vi "力特性判定.vi"(0 "曲线引用":refnum<vi>, 1 "力特性":T1, 3 "错误输入":errorcluster) -> (7 "曲线引用输出":refnum<vi>, 8 "OK？":bool, 10 "错误输出":errorcluster)   [LabVIEW 2018]
uses:
  Global_Variable/Global.vi
  Global_Variable/A180648.vi
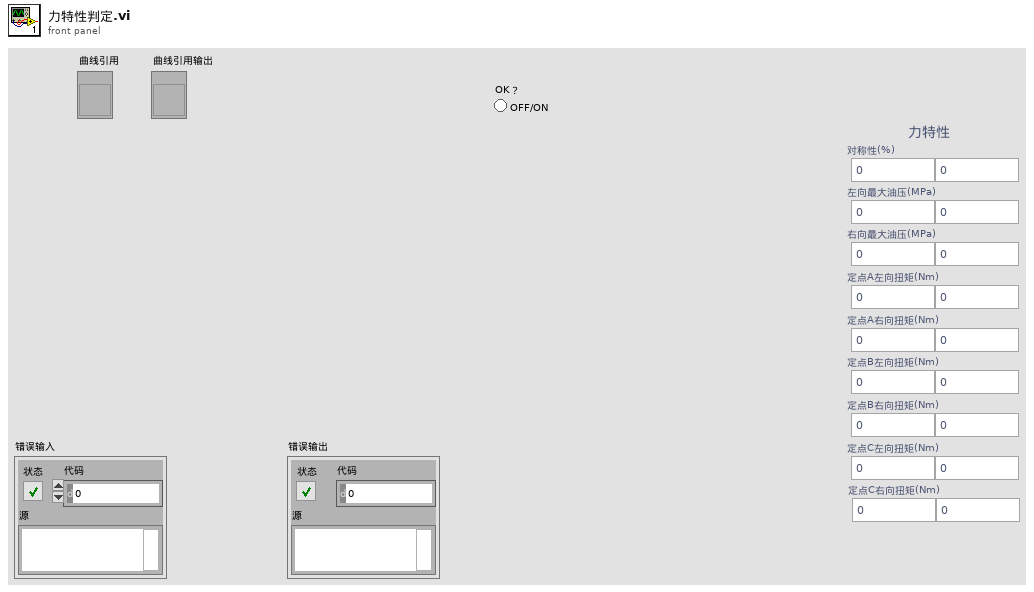
[diagram p1: front panel]
types:
  T1 = cluster{"对称性(%)":cluster{"下限":dbl, "上限":dbl}, "左向最大油压(MPa)":cluster{"下限":dbl, "上限":dbl}, "右向最大油压(MPa)":cluster{"下限":dbl, "上限":dbl}, "定点A左向扭矩(Nm)":cluster{"下限":dbl, "上限":dbl}, "定点A右向扭矩(Nm)":cluster{"下限":dbl, "上限":dbl}, "定点B左向扭矩(Nm)":cluster{"下限":dbl, "上限":dbl}, "定点B右向扭矩(Nm)":cluster{"下限":dbl, "上限":dbl}, "定点C左向扭矩(Nm)":cluster{"下限":dbl, "上限":dbl}, "定点C右向扭矩(Nm)":cluster{"下限":dbl, "上限":dbl}}
  T2 = enum32{"空载", "功能", "力特性", "传感器特性", "电流特性", "振动NVH", "逆向空载", "完成"}
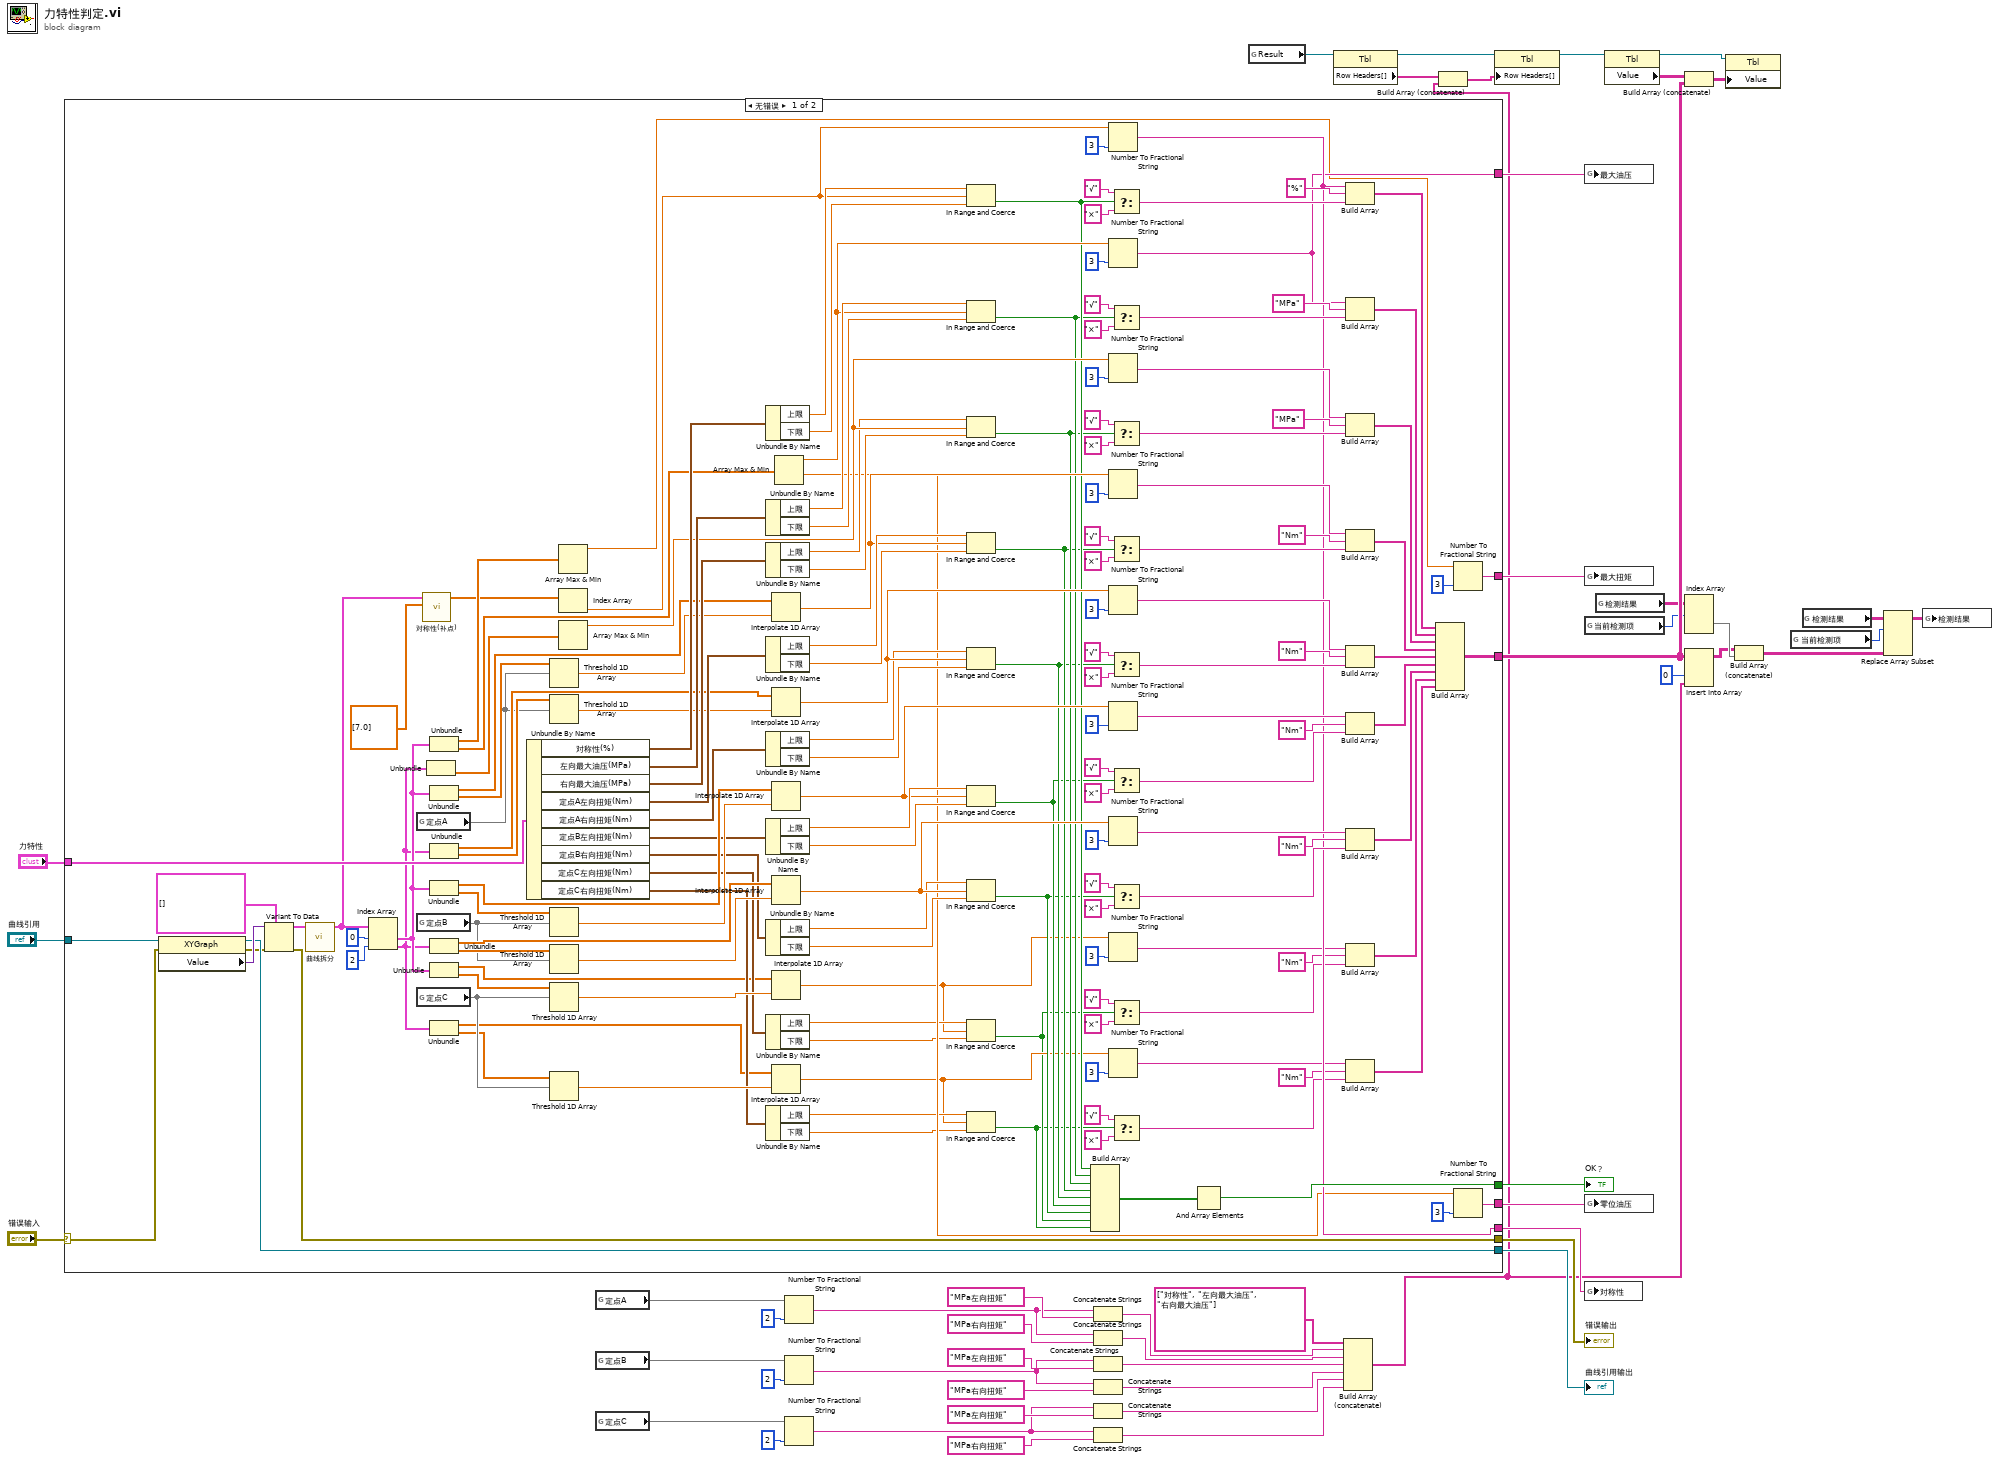
[diagram p0: block diagram]
diagram:
  n1 = case shown="无错误" "错误输入" {
    selector: "错误输入" -> [w206 w210]
    tunnel: [w203 w210] -> w50
    tunnel: "曲线引用" -> [w202 w209]
    tunnel: [w205 w209] -> w48
    tunnel: [w104 _] -> w47
    tunnel: "力特性" -> [w201 _]
    tunnel: [w103 _] -> w10
    tunnel: [w98 _] -> w25
    tunnel: [w97 _] -> w24
    tunnel: [w93 _] -> w23
    tunnel: [w90 _] -> w22
    frame No Error {
      n2 = property class="XYGraph"(reference=w202, error in=w206) -> (reference out=w205:refnum<vi>, error out=w204:errorcluster, "Value"=w208:variant)
      n3 = Variant To Data(error in=w204, type=cluster{dbl[], dbl[]}[] [], Variant=w208) -> (data=w56:cluster{dbl[], dbl[]}[], error out=w203:errorcluster)
      n4 = call "曲线拆分.vi"("原始曲线"=w56) -> ("拆分后曲线"=w55:cluster{dbl[], dbl[]}[])  [unwired: 10 in]
      n5 = Index Array(array=w55, index #1=0 ("索引"), index #2=2 ("索引")) -> (element #1=w70:cluster{dbl[], dbl[]}, element #2=w69:cluster{dbl[], dbl[]})
      n6 = global read "A180648.vi" "定点A"() -> (w100)
      n7 = global read "A180648.vi" "定点B"() -> (w99)
      n8 = global read "A180648.vi" "定点C"() -> (w65)
      n9 = call "对称性(补点).vi"("检测点"=dbl[] [7.0], "XY图"=w55) -> ("对称性"=w53:dbl[])  [unwired: 9 in]
      n10 = Unbundle(w69) -> (w101:dbl[])  [unwired: 1 out]
      n11 = Unbundle(w70) -> (w96:dbl[], w102:dbl[])
      n12 = Unbundle(w70) -> (w164:dbl[], w165:dbl[])
      n13 = Unbundle(w69) -> (w158:dbl[], w157:dbl[])
      n14 = Unbundle(w70) -> (w138:dbl[], w139:dbl[])
      n15 = Unbundle(w69) -> (w130:dbl[], w129:dbl[])
      n16 = Unbundle(w70) -> (w61:dbl[], w66:dbl[])
      n17 = Unbundle(w69) -> (w62:dbl[], w64:dbl[])
      n18 = Unbundle By Name(w201) -> ("对称性(%)"=w200:cluster{"下限":dbl, "上限":dbl}, "左向最大油压(MPa)"=w185:cluster{"下限":dbl, "上限":dbl}, "右向最大油压(MPa)"=w174:cluster{"下限":dbl, "上限":dbl}, "定点A左向扭矩(Nm)"=w161:cluster{"下限":dbl, "上限":dbl}, "定点A右向扭矩(Nm)"=w148:cluster{"下限":dbl, "上限":dbl}, "定点B左向扭矩(Nm)"=w133:cluster{"下限":dbl, "上限":dbl}, "定点B右向扭矩(Nm)"=w120:cluster{"下限":dbl, "上限":dbl}, "定点C左向扭矩(Nm)"=w68:cluster{"下限":dbl, "上限":dbl}, "定点C右向扭矩(Nm)"=w67:cluster{"下限":dbl, "上限":dbl})
      n19 = Threshold 1D Array(2:w100, 3:w165) -> (0:w163:dbl)  [unwired: 1 in]
      n20 = Threshold 1D Array(2:w100, 3:w157) -> (0:w159:dbl)  [unwired: 1 in]
      n21 = Threshold 1D Array(2:w99, 3:w139) -> (0:w137:dbl)  [unwired: 1 in]
      n22 = Threshold 1D Array(2:w99, 3:w129) -> (0:w131:dbl)  [unwired: 1 in]
      n23 = Threshold 1D Array(2:w65, 3:w66) -> (0:w71:dbl)  [unwired: 1 in]
      n24 = Threshold 1D Array(2:w65, 3:w64) -> (0:w81:dbl)  [unwired: 1 in]
      n25 = Array Max & Min(array=w96) -> (max value=w94:dbl)  [unwired: 3 out]
      n26 = Index Array(array=w53) -> (element=w52:dbl)  [unwired: 1 in]
      n27 = Array Max & Min(array=w101) -> (max value=w183:dbl)  [unwired: 3 out]
      n28 = Unbundle By Name(w200) -> ("上限"=w199:dbl, "下限"=w198:dbl)
      n29 = Unbundle By Name(w185) -> ("上限"=w186:dbl, "下限"=w187:dbl)
      n30 = Unbundle By Name(w174) -> ("上限"=w182:dbl, "下限"=w181:dbl)
      n31 = Unbundle By Name(w161) -> ("上限"=w166:dbl, "下限"=w167:dbl)
      n32 = Unbundle By Name(w148) -> ("上限"=w156:dbl, "下限"=w155:dbl)
      n33 = Unbundle By Name(w133) -> ("上限"=w140:dbl, "下限"=w141:dbl)
      n34 = Unbundle By Name(w120) -> ("上限"=w128:dbl, "下限"=w127:dbl)
      n35 = Unbundle By Name(w68) -> ("上限"=w72:dbl, "下限"=w73:dbl)
      n36 = Unbundle By Name(w67) -> ("上限"=w82:dbl, "下限"=w83:dbl)
      n37 = Interpolate 1D Array(1:w163, 2:w164) -> (0:w162:dbl)
      n38 = Interpolate 1D Array(1:w159, 2:w158) -> (0:w160:dbl)
      n39 = Interpolate 1D Array(1:w137, 2:w138) -> (0:w136:dbl)
      n40 = Interpolate 1D Array(1:w131, 2:w130) -> (0:w132:dbl)
      n41 = Interpolate 1D Array(1:w71, 2:w61) -> (0:w63:dbl)
      n42 = Interpolate 1D Array(1:w81, 2:w62) -> (0:w80:dbl)
      n43 = Array Max & Min(array=w102) -> (max value=w184:dbl, min value=w91:dbl)  [unwired: 2 out]
      n44 = In Range and Coerce(upper limit=w199, x=w52, lower limit=w198) -> (In Range?=w118:bool)  [unwired: 1 out]
      n45 = In Range and Coerce(upper limit=w186, x=w184, lower limit=w187) -> (In Range?=w116:bool)  [unwired: 1 out]
      n46 = In Range and Coerce(upper limit=w182, x=w183, lower limit=w181) -> (In Range?=w114:bool)  [unwired: 1 out]
      n47 = In Range and Coerce(upper limit=w166, x=w162, lower limit=w167) -> (In Range?=w112:bool)  [unwired: 1 out]
      n48 = In Range and Coerce(upper limit=w156, x=w160, lower limit=w155) -> (In Range?=w110:bool)  [unwired: 1 out]
      n49 = In Range and Coerce(upper limit=w140, x=w136, lower limit=w141) -> (In Range?=w108:bool)  [unwired: 1 out]
      n50 = In Range and Coerce(upper limit=w128, x=w132, lower limit=w127) -> (In Range?=w106:bool)  [unwired: 1 out]
      n51 = In Range and Coerce(upper limit=w72, x=w63, lower limit=w73) -> (In Range?=w58:bool)  [unwired: 1 out]
      n52 = In Range and Coerce(upper limit=w82, x=w80, lower limit=w83) -> (In Range?=w57:bool)  [unwired: 1 out]
      n53 = Build Array(w118, w116, w114, w112, w110, w108, w106, w58, w57) -> (w105:bool[])
      n54 = Number To Fractional String(number=w52, precision (6)=i16 3 ("精度(6)")) -> (F-format string=w98:string)  [unwired: 2 in]
      n55 = Number To Fractional String(number=w184, precision (6)=i16 3 ("精度(6)")) -> (F-format string=w97:string)  [unwired: 2 in]
      n56 = Number To Fractional String(number=w183, precision (6)=i16 3 ("精度(6)")) -> (F-format string=w179:string)  [unwired: 2 in]
      n57 = Number To Fractional String(number=w162, precision (6)=i16 3 ("精度(6)")) -> (F-format string=w169:string)  [unwired: 2 in]
      n58 = Number To Fractional String(number=w160, precision (6)=i16 3 ("精度(6)")) -> (F-format string=w153:string)  [unwired: 2 in]
      n59 = Number To Fractional String(number=w136, precision (6)=i16 3 ("精度(6)")) -> (F-format string=w143:string)  [unwired: 2 in]
      n60 = Number To Fractional String(number=w132, precision (6)=i16 3 ("精度(6)")) -> (F-format string=w125:string)  [unwired: 2 in]
      n61 = Number To Fractional String(number=w63, precision (6)=i16 3 ("精度(6)")) -> (F-format string=w78:string)  [unwired: 2 in]
      n62 = Number To Fractional String(number=w80, precision (6)=i16 3 ("精度(6)")) -> (F-format string=w85:string)  [unwired: 2 in]
      n63 = Select(t="√" ("元素"), s=w118, f="×" ("元素")) -> (s? t:f=w193:string)
      n64 = Select(t="√" ("元素"), s=w116, f="×" ("元素")) -> (s? t:f=w192:string)
      n65 = Select(t="√" ("元素"), s=w114, f="×" ("元素")) -> (s? t:f=w175:string)
      n66 = Select(t="√" ("元素"), s=w112, f="×" ("元素")) -> (s? t:f=w173:string)
      n67 = Select(t="√" ("元素"), s=w110, f="×" ("元素")) -> (s? t:f=w149:string)
      n68 = Select(t="√" ("元素"), s=w108, f="×" ("元素")) -> (s? t:f=w147:string)
      n69 = Select(t="√" ("元素"), s=w106, f="×" ("元素")) -> (s? t:f=w121:string)
      n70 = Select(t="√" ("元素"), s=w58, f="×" ("元素")) -> (s? t:f=w74:string)
      n71 = Select(t="√" ("元素"), s=w57, f="×" ("元素")) -> (s? t:f=w89:string)
      n72 = And Array Elements(Boolean array=w105) -> (logical AND=w104:bool)
      n73 = Build Array(w98, "%" ("元素"), w193) -> (w119:string[])
      n74 = Build Array(w97, "MPa" ("元素"), w192) -> (w117:string[])
      n75 = Build Array(w179, "MPa" ("元素"), w175) -> (w115:string[])
      n76 = Build Array(w169, "Nm" ("元素"), w173) -> (w113:string[])
      n77 = Build Array(w153, "Nm" ("元素"), w149) -> (w111:string[])
      n78 = Build Array(w143, "Nm" ("元素"), w147) -> (w109:string[])
      n79 = Build Array(w125, "Nm" ("元素"), w121) -> (w107:string[])
      n80 = Build Array(w78, "Nm" ("元素"), w74) -> (w60:string[])
      n81 = Build Array(w85, "Nm" ("元素"), w89) -> (w59:string[])
      n82 = Build Array(w119, w117, w115, w113, w111, w109, w107, w60, w59) -> (w103:string[][])
      n83 = Number To Fractional String(number=w94, precision (6)=i16 3 ("精度(6)")) -> (F-format string=w93:string)  [unwired: 2 in]
      n84 = Number To Fractional String(number=w91, precision (6)=i16 3 ("精度(6)")) -> (F-format string=w90:string)  [unwired: 2 in]
    }
    frame Error {
    }
  }
  "错误输出" <- w50
  "曲线引用输出" <- w48
  "OK？" <- w47
  n85 = global read "A180648.vi" "定点A"() -> (w39)
  n86 = global read "A180648.vi" "定点B"() -> (w38)
  n87 = global read "A180648.vi" "定点C"() -> (w16)
  n88 = Number To Fractional String(number=w39, precision (6)=i16 2 ("精度(6)")) -> (F-format string=w36:string)  [unwired: 2 in]
  n89 = Number To Fractional String(number=w38, precision (6)=i16 2 ("精度(6)")) -> (F-format string=w33:string)  [unwired: 2 in]
  n90 = Number To Fractional String(number=w16, precision (6)=i16 2 ("精度(6)")) -> (F-format string=w18:string)  [unwired: 2 in]
  n91 = Concatenate Strings(w36, "MPa左向扭矩") -> (w31:string)
  n92 = Concatenate Strings(w36, "MPa右向扭矩") -> (w30:string)
  n93 = Concatenate Strings(w33, "MPa左向扭矩") -> (w29:string)
  n94 = Concatenate Strings(w33, "MPa右向扭矩") -> (w28:string)
  n95 = Concatenate Strings(w18, "MPa左向扭矩") -> (w15:string)
  n96 = Concatenate Strings(w18, "MPa右向扭矩") -> (w14:string)
  n97 = global read "Global.vi" "Result"() -> (w43:refnum<vi>)
  n98 = property class="Tbl"(reference=w43) -> (reference out=w42:refnum<vi>, "Row Headers[]"=w8:string[])  [unwired: 1 in, 1 out]
  n99 = Build Array (concatenate)(string[] ["对称性", "左向最大油压", "右向最大油压"] ("列首字符串[]"), w31, w30, w29, w28, w15, w14) -> (w6:string[])
  n100 = Build Array (concatenate)(w8, w6) -> (w7:string[])
  n101 = property class="Tbl"(reference=w42, "Row Headers[]"=w7) -> (reference out=w41:refnum<vi>)  [unwired: 1 in, 1 out]
  n102 = global write "检测结果.vi" "最大油压"(w24) -> ()
  n103 = global write "检测结果.vi" "最大扭矩"(w23) -> ()
  n104 = global read "A180648.vi" "当前检测项"() -> (w4:T2)
  n105 = global write "检测结果.vi" "零位油压"(w22) -> ()
  n106 = global write "检测结果.vi" "对称性"(w25) -> ()
  n107 = global read "A180648.vi" "检测结果"() -> (w5:string[][][])
  n108 = property class="Tbl"(reference=w41) -> (reference out=w46:refnum<vi>, "Value"=w45:string[][])  [unwired: 1 in, 1 out]
  n109 = Build Array (concatenate)(w45, w10) -> (w44:string[][])
  n110 = Index Array(array=w5, index (dim 0)=w4) -> (element=w2:string[][])  [unwired: 2 in]
  n111 = Insert Into Array(array=w10, index (col)=0 ("禁用的索引 (列)"), new element=w6) -> (w1:string[][])  [unwired: 1 in]
  n112 = property class="Tbl"(reference=w46, "Value"=w44) -> ()  [unwired: 1 in, 2 out]
  n113 = Build Array (concatenate)(w1, w2) -> (w3:string[][])
  n114 = global read "A180648.vi" "当前检测项"() -> (w12:T2)
  n115 = global read "A180648.vi" "检测结果"() -> (w13:string[][][])
  n116 = Replace Array Subset(array=w13, new element=w3, index (dim 0)=w12) -> (w11:string[][][])  [unwired: 2 in]
  n117 = global write "A180648.vi" "检测结果"(w11) -> ()
